vi "Timeout.vi"(8 "error in (no error)":errorcluster, 11 "cRIO Vacuum in":refnum<class "cRIO Vacuum.lvclass">) -> (0 "error out":errorcluster, 3 "cRIO Vacuum out":refnum<class "cRIO Vacuum.lvclass">)   [LabVIEW 2015, in "cRIO-Carbondioxide.lvlib" / "CO2-Actor.lvlib" / "cRIO Vacuum.lvclass"]
uses:
  cRIO Vacuum.lvclass
  CO2 Actor/CO2 Actor.lvclass
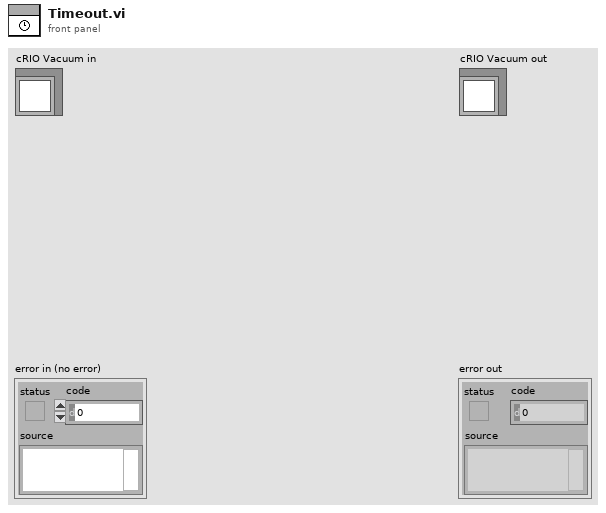
[diagram p1: front panel]
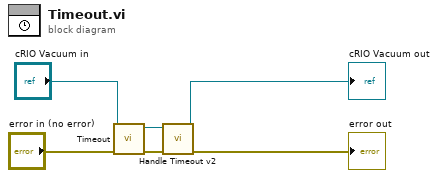
[diagram p0: block diagram]
diagram:
  n1 = call-parent "Timeout.vi"("error in (no error)"="error in (no error)", "CO2 Actor in"="cRIO Vacuum in") -> ("error out"=w4:errorcluster, "CO2 Actor out"=w3:refnum<class "cRIO Vacuum.lvclass">)  [unwired: 8 in]
  n2 = call "Handle Timeout v2.vi"("error in (no error)"=w4, "cRIO Vacuum in"=w3) -> ("error out"=→"error out":errorcluster, "cRIO Vacuum out"=→"cRIO Vacuum out":refnum<class "cRIO Vacuum.lvclass">)  [unwired: 8 in]
